vi "Set Processes Configuration.vi"(10 "Process Settings":T1, 11 "Assembler in":refnum<class "Assembler.lvclass">) -> (3 "Assembler out":refnum<class "Assembler.lvclass">)   [LabVIEW 2019, in "TimingDRV Engine.lvlib" / "Assembler.lvclass"]
uses:
  Assembler.lvclass
  TypeDefs/Process Configuration.ctl
  Assembler.lvclass/Assembler.ctl
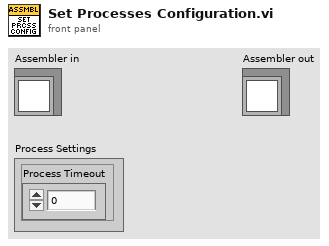
[diagram p1: front panel]
types:
  T1 = typedef "TimingDRV Engine.lvlib/Assembler.lvclass/Process Configuration.ctl" = cluster{"Process Timeout":dbl}
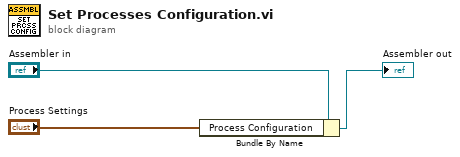
[diagram p0: block diagram]
diagram:
  n1 = Bundle By Name(cluster="Assembler in", "Process Configuration"="Process Settings") -> (→"Assembler out":refnum<class "Assembler.lvclass">)
